vi "Configure Trigger Slope.vi"(8 "error in (no error)":errorcluster, 9 "Trigger Slope (0: Rising)":u16(ring) items=["Positive", "Negative", "Window"], 10 "Channel (1: Channel 1)":u16(ring)=1 items=["Channel 1"=1, "Channel 2"=2, "Channel 3"=3, "Channel 4"=4, "EX"=5, "EX5"=6, "AC Line"=7], 11 "VISA resource name":refnum<visa-resource-name>) -> (0 "error out":errorcluster, 3 "VISA resource name out":refnum<visa-resource-name>)   [LabVIEW 2021, in "Siglent SDS 1000 2000 Series.lvlib"]
doc: "Sets the trigger slope of the specified trigger source."
uses:
  <instrlib>/Siglent SDS 1000 2000 Series/Siglent SDS 1000 2000 Series.lvlib
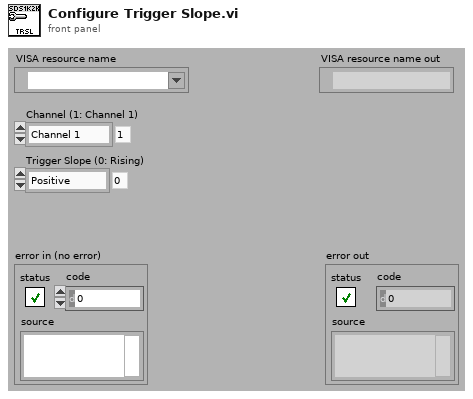
[diagram p1: front panel]
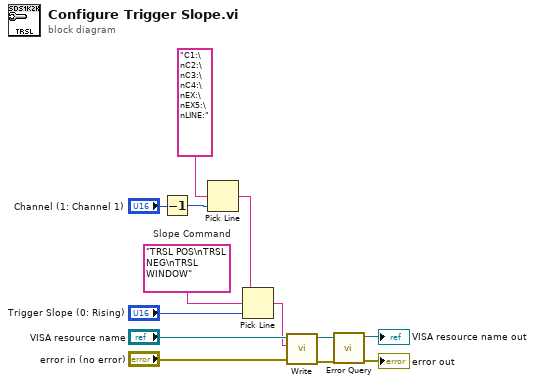
[diagram p0: block diagram]
diagram:
  w13 = "TRSL POS\nTRSL NEG\nTRSL WINDOW"  # Slope Command
  n1 = Decrement(x="Channel (1: Channel 1)") -> (x-1=w1:u16)
  n2 = Pick Line(multi-line string="C1:\nC2:\nC3:\nC4:\nEX:\nEX5:\nLINE:", line index=w1) -> (output string=w8:string)  [unwired: 1 in]
  n3 = Pick Line(string ("")=w8, multi-line string=w13, line index="Trigger Slope (0: Rising)") -> (output string=w7:string)
  n4 = call <instrlib>:"Write.vi"("error in (no error)"="error in (no error)", "Write Buffer"=w7, "VISA resource name"="VISA resource name") -> ("error out"=w3:errorcluster, "VISA resource name out"=w6:refnum<visa-resource-name>)  [unwired: 6 in, 1 out]
  n5 = call <instrlib>:"Error Query.vi"("error in (no error)"=w3, "VISA resource name"=w6) -> ("error out"=→"error out":errorcluster, "VISA resource name out"=→"VISA resource name out":refnum<visa-resource-name>)  [unwired: 6 in, 2 out]
